vi "Classes Construction.vi"(6 "class":T1, 7 "error in":errorcluster, 8 "param2":variant, 9 "param1":variant, 10 "classes in":T2) -> (0 "error out":errorcluster, 2 "init?":bool, 3 "classes out":T2)   [LabVIEW 2011]
uses:
  Controls/Class Objects.ctl
  Modules/File/Configuration/Configuration.lvclass
  Modules/Hardware/Power Supply/Power Supply.lvclass
  Modules/Hardware/Mass Flow Controller/Mass Flow Controller.lvclass
  Modules/File/TDMS/TDMS.lvclass
  Controls/Class Labels.ctl
  Functional Globals/Device Parameters.ctl
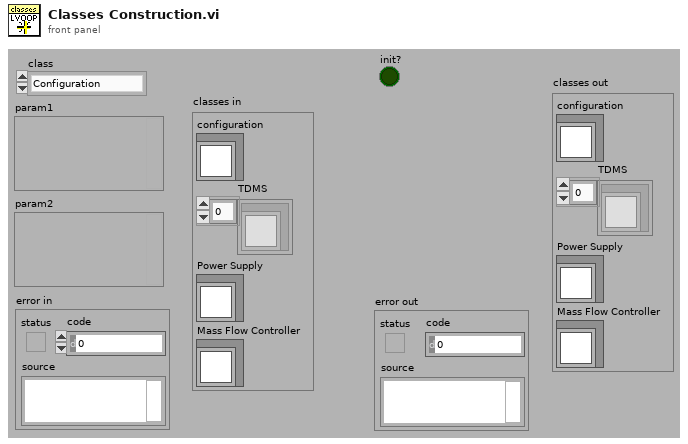
[diagram p1: front panel]
types:
  T1 = typedef "Class Labels.ctl" = enum16{"Configuration", "TDMS", "PID", "Power Supply", "Vapour Generator", "MFC", "NMR", "Valve Controller", "Multimeter"}
  T2 = typedef "Class Objects.ctl" = cluster{"configuration":refnum<class "Configuration.lvclass">, "TDMS":refnum<class "TDMS.lvclass">[], "Power Supply":refnum<class "Power Supply.lvclass">, "Mass Flow Controller":refnum<class "Mass Flow Controller.lvclass">}
  T3 = typedef "Device Parameters.ctl" = enum16{"Initialize", "Set Device Connections", "Set Device Settings", "Get Device Connections", "Get Device Settings"}
  T4 = typedef "Device Settings.ctl" = cluster{"Device Name":cluster{"Setpoint":dbl}}
  T5 = typedef "Device Connections.ctl" = cluster{"Device Name":cluster{"VISA resource name":refnum<visa-resource-name>}}
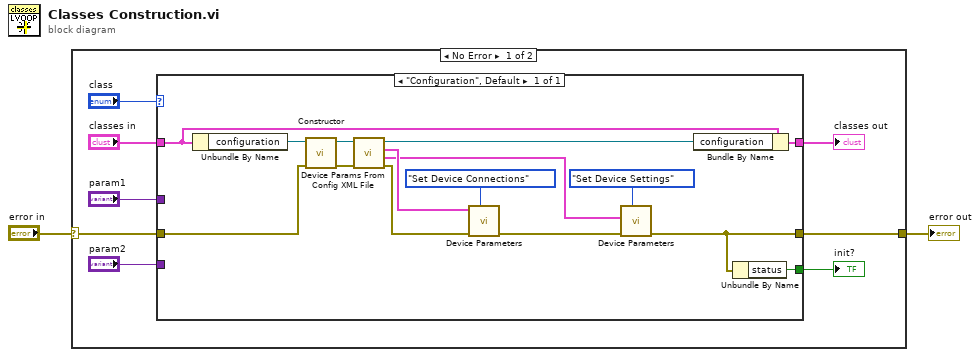
[diagram p0: block diagram]
diagram:
  n1 = case shown="No Error" "error in" {
    selector: "error in" -> [w6 w26]
    tunnel: [w4 w26] -> w1
    frame No Error {
      n2 = case shown="\"Configuration\", Default" "class" {
        tunnel: "classes in" -> [w25]
        tunnel: "param1" -> [_]
        tunnel: "param2" -> [_]
        tunnel: w6 -> [w21]
        tunnel: [w11] -> w4
        tunnel: [w24] -> w5
        tunnel: [w22] -> w3
        frame "Configuration", Default {
          n3 = Unbundle By Name(w25) -> ("configuration"=w23:refnum<class "Configuration.lvclass">)
          n4 = call-dynamic "Constructor.vi"("error in (no error)"=w21, "Configuration in"=w23) -> ("error out"=w19:errorcluster, "Configuration out"=w20:refnum<class "Configuration.lvclass">)  [unwired: 8 in]
          n5 = call "Device Params From Config XML File.vi"("error IN"=w19, "Configuration in"=w20) -> ("error OUT"=w14:errorcluster, "Device Settings"=w12:T4, "Device Connections"=w16:T5, "Configuration out"=w18:refnum<class "Configuration.lvclass">)  [unwired: 6 in]
          n6 = call "Device Parameters.vi"("command"=Device_Parameters."Set Device Connections", "error in"=w14, "Device Connections IN"=w16) -> ("error out"=w13:errorcluster)  [unwired: 6 in, 2 out]
          n7 = call "Device Parameters.vi"("command"=Device_Parameters."Set Device Settings", "error in"=w13, "Device Settings IN"=w12) -> ("error out"=w11:errorcluster)  [unwired: 6 in, 2 out]
          n8 = Bundle By Name(cluster=w25, "configuration"=w18) -> (w24:T2)
          n9 = Unbundle By Name(w11) -> ("status"=w22:bool)
        }
      }
      "init?" <- w3
      "classes out" <- w5
    }
    frame Error {
    }
  }
  "error out" <- w1
